vi "Test Criteria, Record Result, Array.vi"(6 "row (0)":u32, 8 "error in":errorcluster, 10 "Results":dbl[](array[numeric]) format="%.3g", 11 "Tbl Refnum":refnum<vi>) -> (0 "error out":errorcluster, 3 "Tbl Refnum out":refnum<vi>, 4 "row+n":u32)   [LabVIEW 2010]
doc: "This function records results in a Test Criteria table and marks them pass or fail."
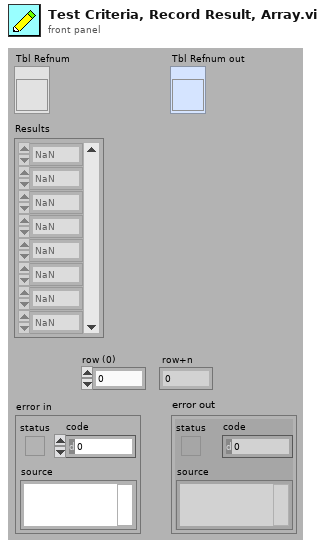
[diagram p1: front panel]
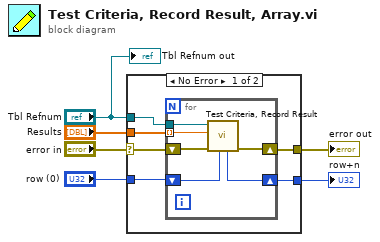
[diagram p0: block diagram]
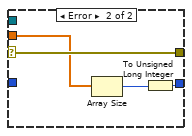
[diagram p2: hidden frame]
diagram:
  n1 = case shown="No Error" "error in" {
    selector: "error in" -> [w11 w22]
    tunnel: [w12 w22] -> w6
    tunnel: "Tbl Refnum" -> [w9 _]
    tunnel: "row (0)" -> [w8 _]
    tunnel: "Results" -> [w10 w21]
    tunnel: [w7 w19] -> w1
    frame No Error {
      n2 = for {
        shift-right: [w17] -> w12
        shift-left: w11 -> [w18]
        tunnel: w10 -> [w16] mode=indexing
        tunnel: w9 -> [w15]
        shift-right: [w13] -> w7
        shift-left: w8 -> [w14]
        n3 = call "Test Criteria, Record Result.vi"("row (0)"=w14, "error in"=w18, "Result"=w16, "Tbl Refnum"=w15) -> ("error out"=w17:errorcluster, "next row"=w13:u32)  [unwired: 5 in, 1 out]
      }
    }
    frame Error {
      n4 = Array Size(array=w21) -> (size(s)=w20:i32)
      n5 = To Unsigned Long Integer(number=w20) -> (unsigned 32bit integer=w19:u32)
    }
  }
  "error out" <- w6
  "row+n" <- w1
  "Tbl Refnum out" <- "Tbl Refnum"
